vi "MenuHandler.vi"(5 "tree control":refnum<vi>, 7 "main queue":refnum<queue>, 8 "error in":errorcluster, 9 "parameters":variant, 10 "menu string":string, 11 "Scope in":refnum<class "Scope Instrument.lvclass">) -> (0 "error out":errorcluster, 1 "refresh tree?":bool, 2 "Unhandled":bool, 3 "Scope out":refnum<class "Scope Instrument.lvclass">)   [LabVIEW 2025, in "Scope.lvlib" / "Scope Instrument.lvclass"]
doc: "Copyright 2017 National Instruments Corporation\n\nLicensed under the Apache License, Version 2.0 (the \"License\"); you may not use this file except in compliance with the License. You may obtain a copy of the License at http://www.apache.org/licenses/LICENSE-2.0\nUnless required by applicable law or agreed to in writing, software distributed under the License is distributed on an \"AS IS\" BASIS, WITHOUT WARRANTIES OR CONDITIONS OF ANY KIND, either express or implied. See the License for the specific language governing permissions and limitations under the License."
uses:
  Scope Instrument.lvclass
  Scope Instrument.lvclass/Scope Instrument.ctl
  Users/Public/Documents/Sandia National Labs/TSS Plugin/Abstract Engine.lvlibp/Abstract Instrument/Abstract Instrument.lvclass
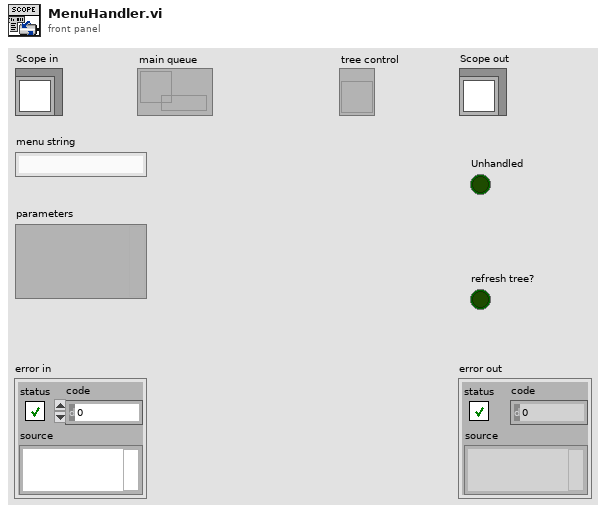
[diagram p1: front panel]
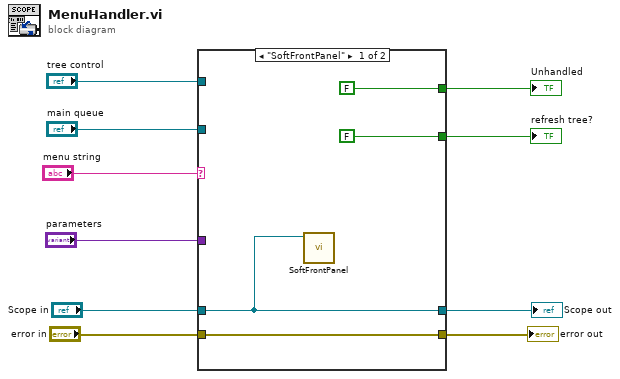
[diagram p0: block diagram]
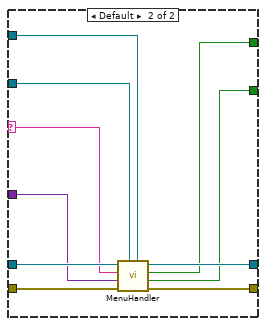
[diagram p2: hidden frame]
diagram:
  n1 = case shown="\"SoftFrontPanel\"" "menu string" {
    selector: "menu string" -> [_ w20]
    tunnel: "error in" -> [w12 w24]
    tunnel: [w12 w23] -> w9
    tunnel: "Scope in" -> [w11 w22]
    tunnel: [w11 w21] -> w6
    tunnel: [FALSE ("Unhandled") w16] -> w5
    tunnel: [FALSE ("refresh tree?") w15] -> w4
    tunnel: "parameters" -> [_ w19]
    tunnel: "main queue" -> [_ w18]
    tunnel: "tree control" -> [_ w17]
    frame "SoftFrontPanel" {
      n2 = call "SoftFrontPanel.vi"("Scope"=w11) -> ()  [unwired: 9 in, 2 out]
    }
    frame Default {
      n3 = call-parent "MenuHandler.vi"("tree control"=w17, "main queue"=w18, "error in"=w24, "parameters"=w19, "menu string"=w20, "CEF_serializable node in"=w22) -> ("error out"=w23:errorcluster, "refresh tree?"=w15:bool, "Unhandled"=w16:bool, "CEF_serializable node out"=w21:refnum<class "Scope Instrument.lvclass">)  [unwired: 2 in]
    }
  }
  "error out" <- w9
  "Scope out" <- w6
  "Unhandled" <- w5
  "refresh tree?" <- w4
